vi "win32 set directory.vi"(8 "error in (no error)":errorcluster, 10 "zValue":u32, 11 "type":u32) -> (0 "error out":errorcluster, 2 "zValue out":u32, 3 "function return":i32)   [LabVIEW 2020, in "sqlite3.lvlib"]
uses:
  sqlite3.lvlib
  errstr.vi
  bin/sqlite3_64.dll
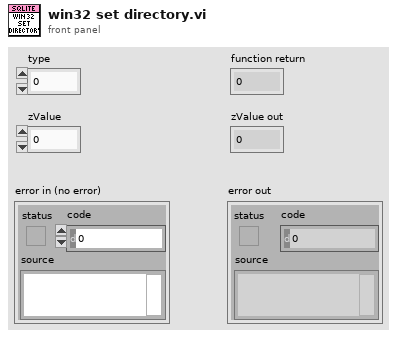
[diagram p1: front panel]
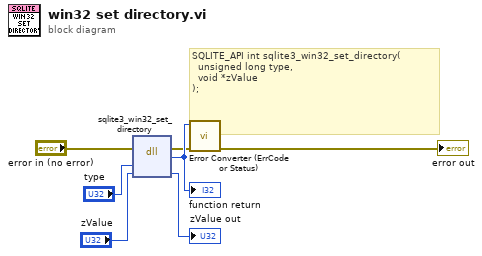
[diagram p0: block diagram]
diagram:
  # "SQLITE_API int sqlite3_win32_set_directory(\n  unsigned long type, \n  void *zValue        \n);"
  n1 = dll-call lib="D:/Project/Labview-Projects/database-configuration/externals/sqlite3/Source/bin/sqlite3_*.*" fn="sqlite3_win32_set_directory"(error in="error in (no error)", "type"="type", "zValue"="zValue") -> (error out=w2:errorcluster, w7:i32, "zValue"=→"zValue out":u32)  [unwired: 3 in, 1 out]
  "function return" <- w7
  n2 = call "Error Converter (ErrCode or Status).vi"("error in (no error)"=w2, "error code"=w7) -> ("error out"=→"error out":errorcluster)  [unwired: 9 in]
